vi "Less Than.vi"(1 "comparable 2":refnum<class "Less Comparable.lvclass">, 2 "comparable 1":refnum<class "Less Comparable.lvclass">) -> (0 "less?":bool)   [LabVIEW 2020, in "Less Comparable.lvclass"]
doc: "Returns whether <b>Comparable 1</b> is less than, equal to, or greater than <b>Comparable 2</b>."
uses:
  <vilib>/Comparison/Less/Less Comparable/Less Comparable.lvclass
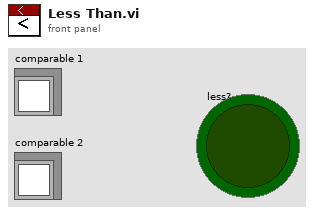
[diagram p1: front panel]
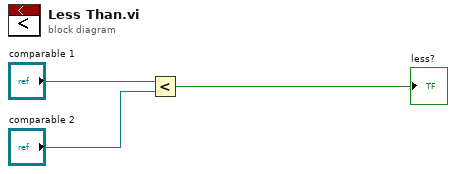
[diagram p0: block diagram]
diagram:
  n1 = Less?(x="comparable 1", y="comparable 2") -> (x < y?=→"less?":bool)
